vi "Generate HeadStatus Event GIS Printer.vi"(8 "error in (no error)":errorcluster, 10 "HeadStatus":T1, 11 "GIS Printer in":refnum<class "GIS Printer.lvclass">) -> (0 "error out":errorcluster, 3 "GIS Printer out":refnum<class "GIS Printer.lvclass">)   [LabVIEW 2022 SP3, in "GIS Printer.lvclass"]
uses:
  GIS Printer.lvclass
  Typedefs/HeadEnableStatus--cluster.ctl
  <vilib>/event_ctls.llb/usereventprio.ctl
  GIS Printer.lvclass/GIS Printer.ctl
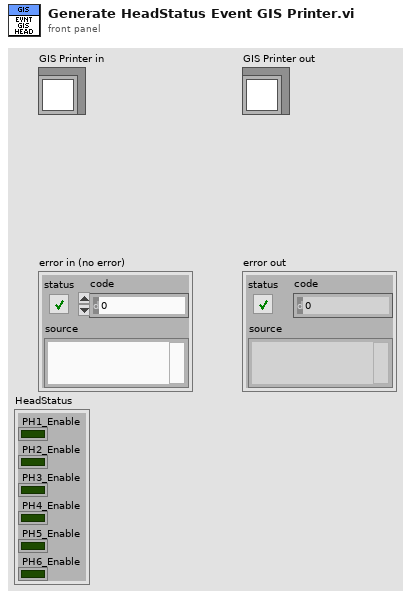
[diagram p1: front panel]
types:
  T1 = typedef "HeadEnableStatus--cluster.ctl" = cluster{"PH1_Enable":bool, "PH2_Enable":bool, "PH3_Enable":bool, "PH4_Enable":bool, "PH5_Enable":bool, "PH6_Enable":bool}
  T2 = typedef "usereventprio.ctl" = enum32{"high priority", "normal priority"}
  T3 = typedef "GIS Printer.lvclass/Private Data.ctl" = cluster{"UserEvents":T4, "All Dependencies":cluster{"Class References":refnum<class>[], "Class Names":string[]}, "PrinterConiguration":T5, "Status":T6, "GISHeadStatus":T7[], "HeadStatus":T1}
  T4 = typedef "GIS Printer.lvclass/UserEvents.ctl" = cluster{"API Incoming Event":refnum<user-event>, "API Executed Event":refnum<user-event>, "API Return Event":refnum<user-event>, "Status Changed Event":refnum<user-event>, "Abort":refnum<user-event>, "stop process":refnum<user-event>, "GISPollStatus":refnum<user-event>, "GISHeadStatus":refnum<user-event>}
  T5 = typedef "GIS Printer.lvclass/PrinterConfiguration--Cluster.ctl" = cluster{"IPAddress":string, "Move Stage on RTP Command?":bool, "Stage Move Position":string, "PH1-Prime Path":path, "PH2-Prime Path":path, "PH3-Prime Path":path, "PH4-Prime Path":path, "PH5-Prime Path":path, "PH6-Prime Path":path, "PrintScriptsFolder":path, "PurgeScriptsFolder":path, "StageScriptsFolder":path, "PH1-HeatOn Path":path, "PH2-HeatOn Path":path, "PH3-HeatOn Path":path, "PH4-HeatOn Path":path, "PH5-HeatOn Path":path, "PH6-HeatOn Path":path, "PH1-HeatOff Path":path, "PH2-HeatOff Path":path, "PH3-HeatOff Path":path, "PH4-HeatOff Path":path, "PH5-HeatOff Path":path, "PH6-HeatOff Path":path}
  T6 = typedef "GIS Printer.lvclass/Status Cluster.ctl" = cluster{"Command Status":variant, "TCP Commands & Responses":string[][], "Printer Busy?":bool}
  T7 = typedef "GIS Status--Cluster.ctl" = cluster{"HeadEnabled":bool, "SpitEnabled":bool, "HeaterEnabled":bool, "TargetTemperature":dbl, "CurrentTemperature":dbl}
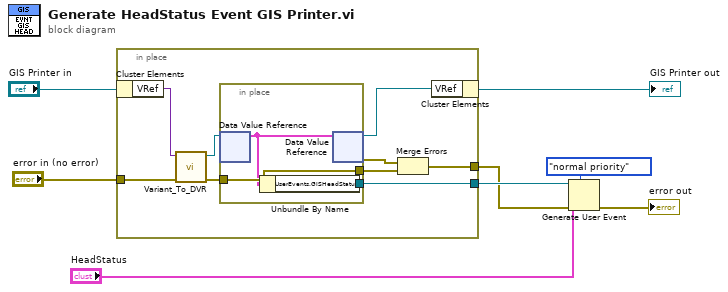
[diagram p0: block diagram]
diagram:
  n1 = in-place {
    in-place-border: [w13] -> w8
    in-place-border: "error in (no error)" -> [w12]
    in-place-border: [w11] -> w5
    n2 = in-place-cluster #1("GIS Printer in") -> ("VRef"=w10:variant)
    n3 = call "Variant_To_DVR.vi"("error in (no error)"=w12, "Variant"=w10) -> ("error out"=w16:errorcluster, "DVR"=w17:refnum<data-value>)  [unwired: 8 in]
    n4 = in-place {
      in-place-border: w16 -> [w20]
      in-place-border: [w20] -> w15
      in-place-border: [w19] -> w13
      n5 = in-place-dvr #2(w17) -> (w18:T3)  [unwired: 1 out]
      n6 = Unbundle By Name(w18) -> ("UserEvents.GISHeadStatus"=w19:refnum<user-event>)
      n7 = in-place-dvr #2(w18) -> (w9:refnum<data-value>, w14:errorcluster)
    }
    n8 = Merge Errors(w14, w15) -> (w11:errorcluster)
    n9 = in-place-cluster #1("VRef"=w9) -> (→"GIS Printer out":refnum<class "GIS Printer.lvclass">)
  }
  n10 = Generate User Event(priority (normal)=usereventprio."normal priority", user event=w8, event data cluster="HeadStatus", error in=w5) -> (error out=→"error out":errorcluster)  [unwired: 1 out]
